vi "Runtest - Deamon Ref (FGV).vi"(6 "Action":T1=enum."Write", 8 "error in":errorcluster, 10 "Name":string[](array[string]), 11 "Ref in":refnum<vi>[](array[refnum])) -> (0 "error out":errorcluster, 2 "Name out":string[](array[string]), 3 "Ref out":refnum<vi>[](array[refnum]))   [LabVIEW 2019]
uses:
  Controls/FGV States.ctl
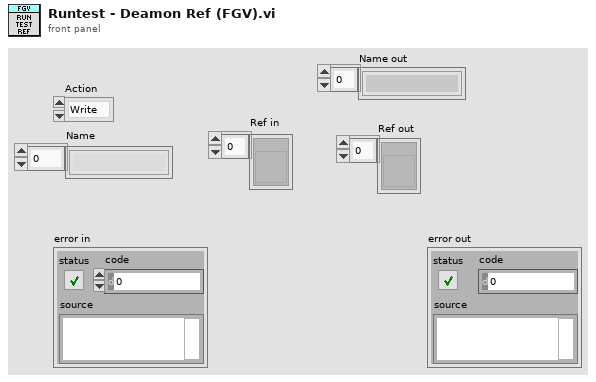
[diagram p1: front panel]
types:
  T1 = typedef "FGV States.ctl" = enum16{"Read", "Write"}
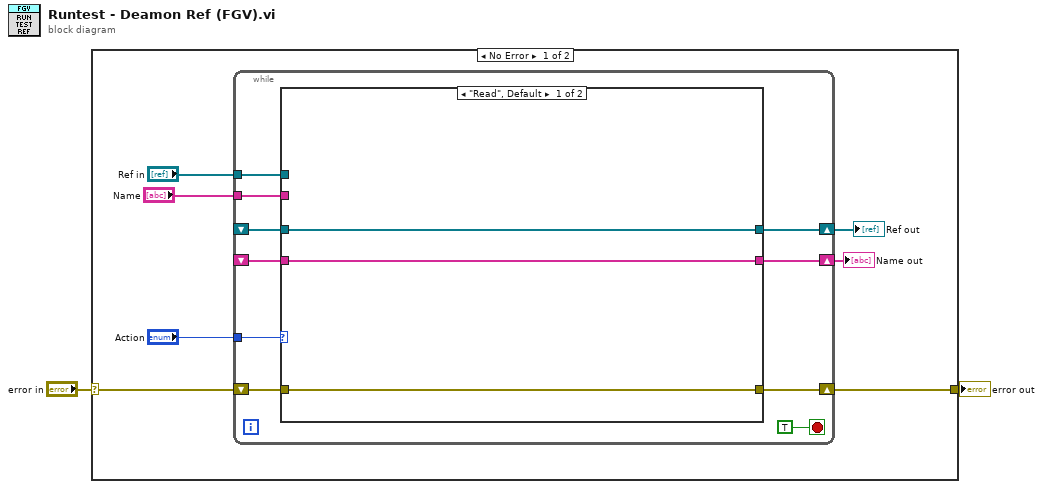
[diagram p0: block diagram]
diagram:
  n1 = case shown="No Error" "error in" {
    selector: "error in" -> [w9 w26]
    tunnel: [w8 w26] -> w1
    frame No Error {
      n2 = while {
        tunnel: "Action" -> [w17]
        shift-right: [w18] -> w8
        shift-left: w9 -> [w19]
        tunnel: "Ref in" -> [w16]
        shift-right: [w15] -> w5
        shift-left: _ -> [w14]
        tunnel: "Name" -> [w12]
        shift-right: [w11] -> w3
        shift-left: _ -> [w10]
        stop <- TRUE stop-if-true
        n3 = case shown="\"Read\", Default" w17 {
          tunnel: w19 -> [w22 w24]
          tunnel: [w22 w24] -> w18
          tunnel: w16 -> [_ w25]
          tunnel: [w21 w25] -> w15
          tunnel: w14 -> [w21 _]
          tunnel: w12 -> [_ w23]
          tunnel: [w20 w23] -> w11
          tunnel: w10 -> [w20 _]
          frame "Read", Default {
          }
          frame "Write" {
          }
        }
      }
      "Ref out" <- w5
      "Name out" <- w3
    }
    frame Error {
    }
  }
  "error out" <- w1
